vi "Timer_FeedbackNode.vi"(7 "Timer action (read)":T1=enum."Read", 8 "error in (no error)":errorcluster) -> (0 "error out":errorcluster, 3 "Numeric":dbl format="%#.2f")   [LabVIEW 2020]
uses:
  #typedef_FGV_TimerAction.ctl
panel:
  out "Time Elapsed?":bool
  in  "TimeToElapse (s)":dbl=10.0
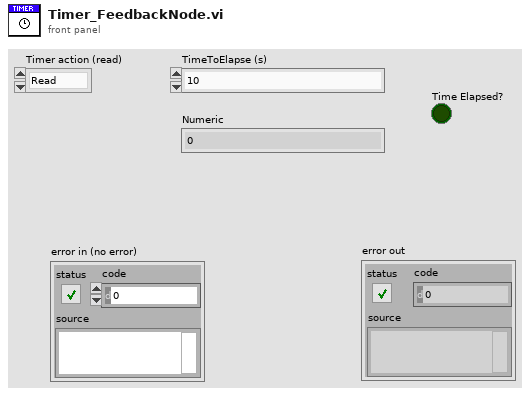
[diagram p1: front panel]
types:
  T1 = typedef "#typedef_FGV_TimerAction.ctl" = enum16{"Reset", "Read"}
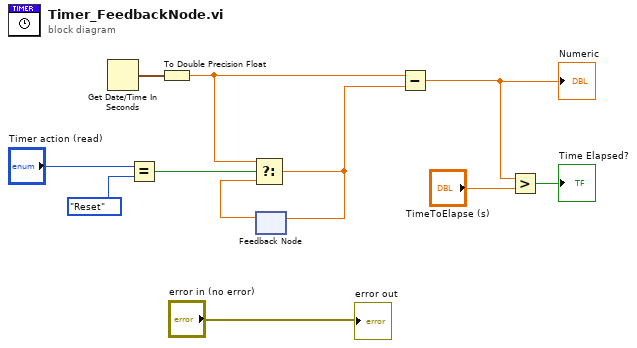
[diagram p0: block diagram]
diagram:
  n1 = Get Date/Time In Seconds() -> (seconds since 1Jan1904=w8:timestamp)
  n2 = Equal?(x="Timer action (read)", y=#typedef_FGV_TimerAction."Reset") -> (x = y?=w2:bool)
  n3 = To Double Precision Float(number=w8) -> (double precision float=w6:dbl)
  n4 = feedback #1() -> (w5:dbl)  [unwired: 1 in]
  n5 = Select(t=w6, s=w2, f=w5) -> (s? t:f=w4:dbl)
  n6 = feedback-in #1(w4) -> ()
  n7 = Subtract(x=w6, y=w4) -> (x-y=w10:dbl)
  "Numeric" <- w10
  n8 = Greater?(x=w10, y="TimeToElapse (s)") -> (0:→"Time Elapsed?":bool)
  "error out" <- "error in (no error)"
